vi "_Raise Navigation Starting Event.vi"(4 "Display State In":T1, 5 "Event Data":cluster{"sender":refnum<k24>, "e":refnum<k24>}, 6 "Control Ref":refnum<k24>, 7 "Event Common Data":T2) -> ()   [LabVIEW 2020, in "WebView2 Control.xctl"]
uses:
  WebView2 Control.xctl
  E:/Labview/LV 2020/Libs/LV-WebView2/microsoft.web.webview2/lib/net45/Microsoft.Web.WebView2.Core.dll
  microsoft.web.webview2/lib/net45/Microsoft.Web.WebView2.Core.dll
  Events.ctl
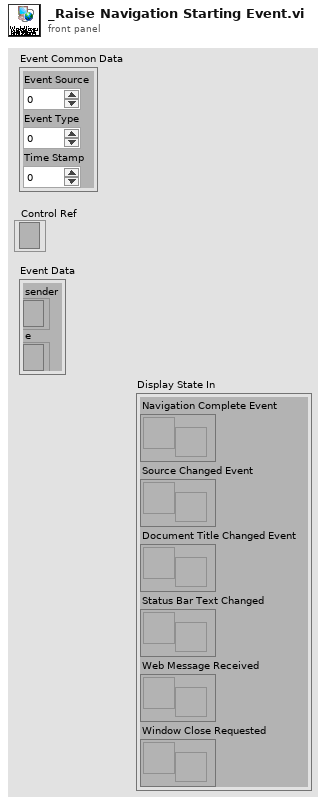
[diagram p1: front panel]
types:
  T1 = typedef "WebView2 Control.xctl/Events.ctl" = cluster{"Navigation Complete Event":refnum<user-event>, "Source Changed Event":refnum<user-event>, "Document Title Changed Event":refnum<user-event>, "Status Bar Text Changed":refnum<user-event>, "Web Message Received":refnum<user-event>, "Window Close Requested":refnum<user-event>}
  T2 = cluster{"Event Source":i32, "Event Type":u32, "Time Stamp":u32}
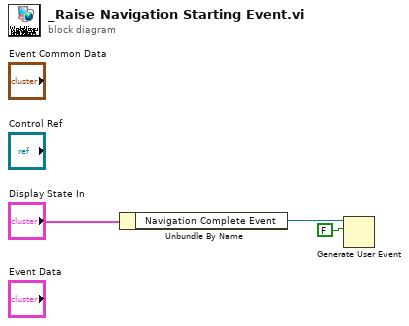
[diagram p0: block diagram]
diagram:
  n1 = Unbundle By Name("Display State In") -> ("Navigation Complete Event"=w3:refnum<user-event>)
  n2 = Generate User Event(user event=w3, event data cluster=FALSE ("event data")) -> ()  [unwired: 2 in, 2 out]
